vi "FileBuffer.vi"(9 "Boolean":bool, 10 "FileDataChannel":T1, 11 "Refnum in":refnum<k33>) -> (3 "# elements":u32)   [LabVIEW 2018]
uses:
  Clusters/FileDataChannel.ctl
panel:
  out "Array":dbl[](array[numeric])
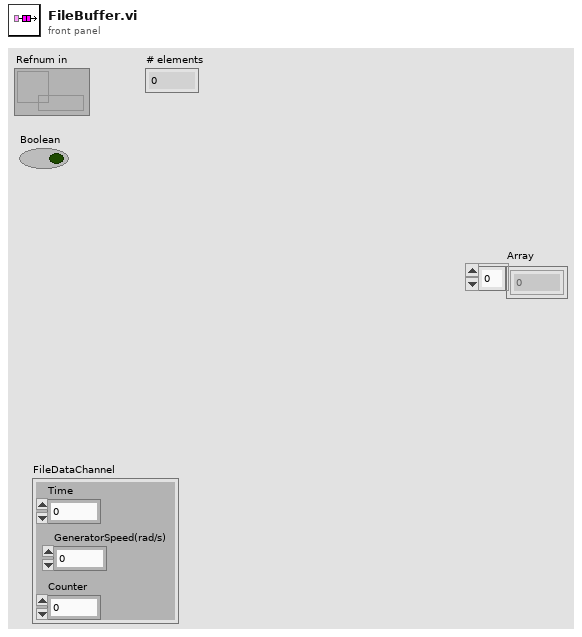
[diagram p1: front panel]
types:
  T1 = typedef "FileDataChannel.ctl" = cluster{"GeneratorSpeed(rad/s)":sgl, "Counter":sgl, "Time":sgl}
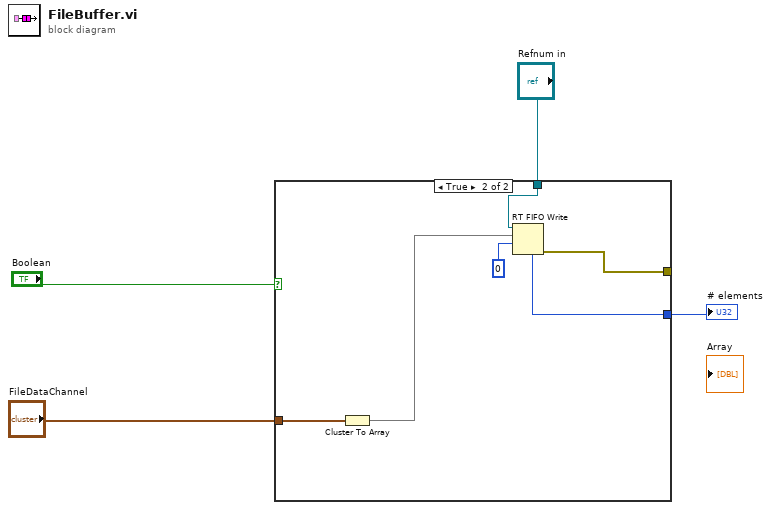
[diagram p0: block diagram]
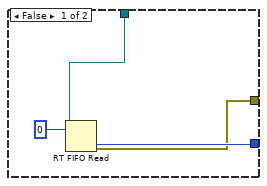
[diagram p2: hidden frame]
diagram:
  n1 = case shown="True" "Boolean" {
    tunnel: "Refnum in" -> [w8 w14]
    tunnel: [w6 w12] -> w3
    tunnel: [w5 w11] -> _
    tunnel: "FileDataChannel" -> [_ w10]
    frame False {
      n2 = RT FIFO Read(0:w8, 2:0) -> (7:w6:u32, 11:w5:errorcluster)  [unwired: 2 in, 3 out]
    }
    frame True {
      n3 = Cluster To Array(cluster=w10) -> (array=w9:sgl[])
      n4 = RT FIFO Write(0:w14, 1:w9, 2:0) -> (7:w12:u32, 11:w11:errorcluster)  [unwired: 2 in, 2 out]
    }
  }
  "# elements" <- w3
